vi "Build_tdms_ch_name.vi"(11 "Event_nb":i32) -> (3 "Channel_name":string[](array[string]))   [LabVIEW 2019]
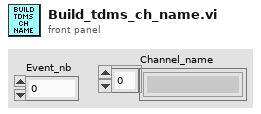
[diagram p1: front panel]
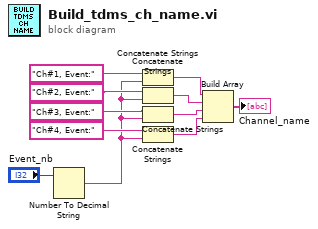
[diagram p0: block diagram]
diagram:
  n1 = Number To Decimal String(number="Event_nb") -> (decimal integer string=w1:string)  [unwired: 1 in]
  n2 = Concatenate Strings("Ch#1, Event:" ("group name in (Untitled)"), w1) -> (w7:string)
  n3 = Concatenate Strings("Ch#2, Event:" ("group name in (Untitled)"), w1) -> (w9:string)
  n4 = Concatenate Strings("Ch#3, Event:" ("group name in (Untitled)"), w1) -> (w10:string)
  n5 = Concatenate Strings("Ch#4, Event:" ("group name in (Untitled)"), w1) -> (w11:string)
  n6 = Build Array(w7, w9, w10, w11) -> (→"Channel_name":string[])
